vi "PH_USB600x_AnalogReader.set trigger mode.vi"(0 "i ref in":refnum<vi>, 1 "triggerSource (\"PFI0\")":string, 2 "edgeRising":bool, 5 "error in (no error)":errorcluster, 7 "triggerType":T1(ring) caption="useExtTrigger", 9 "level":dbl format="%0.2f", 11 "pretriggerSamples":u32=100) -> (14 "i ref out":refnum<vi>, 19 "error out":errorcluster)   [LabVIEW 2014, in "PH_USB600x_AnalogReader.lvlib"]
doc: "Sets the trigger mode for the scope.\n\nLicense Agreement for this software:\n\nCopyright (C)\nGesellschaft für Schwerionenforschung, GSI\nPlanckstr. 1\n64291 Darmstadt\nGermany\n\nContact: D.Beck@gsi.de \n\nThis program is free software; you can redistribute it and/or modify it under the terms of the GNU General Public License as published by the Free Software Foundation; either version 2 of the license, or (at your option) any later version.\n\nThis program is distributed in the hope that it will be useful, but WITHOUT ANY WARRANTY; without even the implied warranty of MERCHANTABILITY or FITNESS FOR A PARTICULAR PURPOSE. See the GNU General License for more details (http://www.gnu.org).\n\nGesellschaft für Schwerionenforschung, GSI\nPlanckstr. 1, 64291 Darmstadt, Germany\nFor all questions and ideas contact: M.Richter@gsi.de, H.Brand@gsi.de or D.Beck@gsi.de.\nLast update: 17-JUN-2004"
uses:
  PH_USB600x_AnalogReader.lvlib
  PH_Basics/PH_StatusHandler/PH_StatusHandler.Status.ctl
  <vilib>/DAQmx/configure/trigger.llb/DAQmx Reference Trigger (None).vi
  <vilib>/DAQmx/configure/trigger.llb/DAQmx Reference Trigger (Analog Edge).vi
  <vilib>/DAQmx/configure/trigger.llb/DAQmx Reference Trigger (Digital Edge).vi
  PH_Basics/PH_StatusHandler/PH_StatusHandler.lvlib
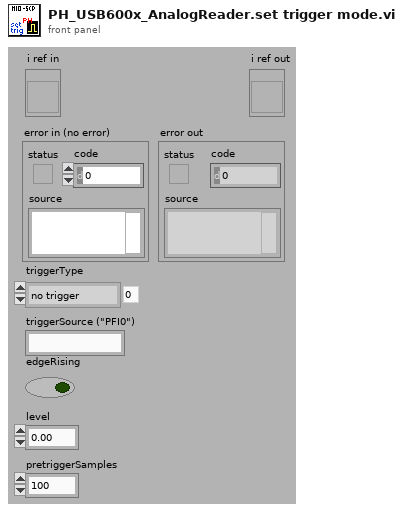
[diagram p1: front panel]
types:
  T1 = enum32{"no trigger", "digital trigger", "analog trigger"}
  T2 = typedef "PH_USB600x_AnalogReader.lvlib/PH_USB600x_AnalogReader.i attribute.ctl" = cluster{"GUI Refs":cluster{"Delete":refnum<vi>, "Status":refnum<vi>, "Timeout":refnum<vi>, "Acquire Waveform":refnum<vi>, "Timing":refnum<vi>, "Graph":refnum<vi>, "Prdc Interval":refnum<vi>, "Formula":refnum<vi>}, "Device Settings":cluster{"AIChannel":refnum<k21>, "channelName":string, "Status":T3}, "Timing":T4, "Prdc Interval":dbl, "Lin Scaling":T5, "Data":cluster{"t0":timestamp, dbl}[]}
  T3 = typedef "PH_StatusHandler.lvlib/PH_StatusHandler.Status.ctl" = i16
  T4 = typedef "PH_USB600x_AnalogReader.lvlib/PH_USB600x_AnalogReader.Timing.ctl" = cluster{"Samples per Channel":i32, "Rate":dbl}
  T5 = typedef "PH_USB600x_AnalogReader.lvlib/PH_USB600x_AnalogReader.Lin Scaling.ctl" = cluster{"Slope [Unit/V]":dbl, "Offset [Unit]":dbl, "Y-Unit":string, "Y-Label":string}
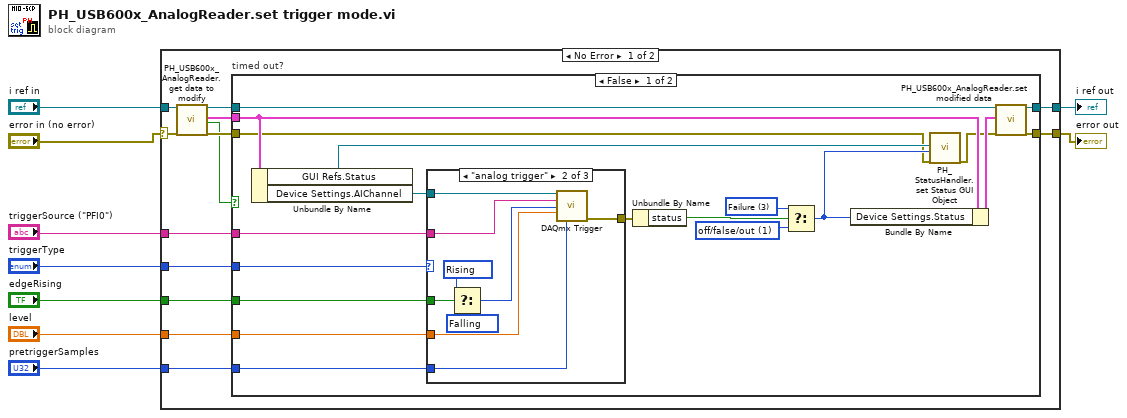
[diagram p0: block diagram]
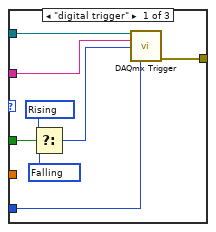
[diagram p2: hidden frame]
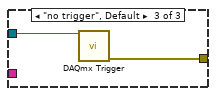
[diagram p3: hidden frame]
diagram:
  n1 = case shown="No Error" "error in (no error)" {
    selector: "error in (no error)" -> [w10 w63]
    tunnel: "i ref in" -> [w22 w64]
    tunnel: [w20 w64] -> w8
    tunnel: [w18 w63] -> w7
    tunnel: "triggerSource (\"PFI0\")" -> [w15 _]
    tunnel: "triggerType" -> [w14 _]
    tunnel: "edgeRising" -> [w13 _]
    tunnel: "level" -> [w12 _]
    tunnel: "pretriggerSamples" -> [w11 _]
    frame No Error {
      n2 = call "PH_USB600x_AnalogReader.get data to modify.vi"("i ref in"=w22, "error in (no error)"=w10) -> ("i ref out"=w21:refnum<vi>, "i attribute"=w16:T2, "timed out"=w17:bool, "error out"=w19:errorcluster)  [unwired: 14 in]
      n3 = case "timed out?" shown="False" w17 {
        tunnel: [w41 w62] -> w20
        tunnel: w21 -> [w35 w62]
        tunnel: [w26 w61] -> w18
        tunnel: w19 -> [w24 w61]
        tunnel: w16 -> [w28 _]
        tunnel: w15 -> [w38 _]
        tunnel: w14 -> [w40 _]
        tunnel: w13 -> [w37 _]
        tunnel: w12 -> [w36 _]
        tunnel: w11 -> [w34 _]
        frame False {
          w31 = T3 1 items=["no info", "off/false/out", "on/true/in", "Failure", "Alarm", "Status 1", "Status 2", "Status 3"] ("Device Settings.Status")
          w32 = T3 3 items=["no info", "off/false/out", "on/true/in", "Failure", "Alarm", "Status 1", "Status 2", "Status 3"] ("Device Settings.Status")
          n4 = Unbundle By Name(w28) -> ("GUI Refs.Status"=w30:refnum<vi>, "Device Settings.AIChannel"=w39:refnum<k21>)
          n5 = case shown="\"analog trigger\"" w40 {
            tunnel: w39 -> [w49 w53 w60]
            tunnel: [w44 w55 w59] -> w29
            tunnel: w38 -> [w43 w52 _]
            tunnel: w37 -> [w48 w58 _]
            tunnel: w36 -> [_ w54 _]
            tunnel: w34 -> [w42 w50 _]
            frame "digital trigger" {
              w46 = 10171 items=["Rising"=10280, "Falling"=10171] ("edge")
              w47 = 10280 items=["Rising"=10280, "Falling"=10171] ("edge")
              n6 = Select(t=w47, s=w48, f=w46) -> (s? t:f=w45:i32)
              n7 = call-poly <vilib>:"DAQmx Trigger.vi"("task/channels in"=w49, "source"=w43, "edge"=w45, "pretrigger samples per channel"=w42) -> ("error out"=w44:errorcluster)  [unwired: 10 in, 1 out]
            }
            frame "analog trigger" {
              w56 = 10171 items=["Rising"=10280, "Falling"=10171] ("edge")
              w57 = 10280 items=["Rising"=10280, "Falling"=10171] ("edge")
              n8 = Select(t=w57, s=w58, f=w56) -> (s? t:f=w51:i32)
              n9 = call-poly <vilib>:"DAQmx Trigger.vi"("task/channels in"=w53, "source"=w52, "slope"=w51, "level"=w54, "pretrigger samples per channel"=w50) -> ("error out"=w55:errorcluster)  [unwired: 9 in, 1 out]
            }
            frame "no trigger", Default {
              n10 = call-poly <vilib>:"DAQmx Trigger.vi"("task/channels in"=w60) -> ("error out"=w59:errorcluster)  [unwired: 13 in, 1 out]
            }
          }
          n11 = Unbundle By Name(w29) -> ("status"=w33:bool)
          n12 = Select(t=w32, s=w33, f=w31) -> (s? t:f=w25:T3)
          n13 = Bundle By Name(cluster=w28, "Device Settings.Status"=w25) -> (w27:T2)
          n14 = call "PH_StatusHandler.set Status GUI Object.vi"("PH Status Ref"=w30, "Value"=w25, "error in (no error)"=w24) -> ("error out"=w23:errorcluster)  [unwired: 16 in]
          n15 = call "PH_USB600x_AnalogReader.set modified data.vi"("i ref in"=w35, "i attribute"=w27, "error in (no error)"=w23) -> ("i ref out"=w41:refnum<vi>, "error out"=w26:errorcluster)  [unwired: 15 in]
        }
        frame True {
        }
      }
    }
    frame Error {
    }
  }
  "error out" <- w7
  "i ref out" <- w8
